vi "Create DigiPattern File_BML.vi"(7 "Timeset between frms":u32=50, 8 "error in (no error)":errorcluster, 9 "Pattern Name":string, 10 "BML Frame Array":refnum<class "BML_Frame_Root.lvclass">[](array[class]), 11 "BML_DigiPattern_Generator.lvclass":refnum<class "DigiPattern_Generator.lvclass">) -> (0 "error out":errorcluster, 3 "BML_DigiPattern_Generator.lvclass out":refnum<class "DigiPattern_Generator.lvclass">)   [LabVIEW 2018, in "DigiPattern_Generator.lvclass"]
uses:
  DigiPattern_Generator.lvclass
  BML_Frame_Root/BML_Frame_Root.lvclass
  DigiPattern_Generator.lvclass/DigiPattern_Generator.ctl
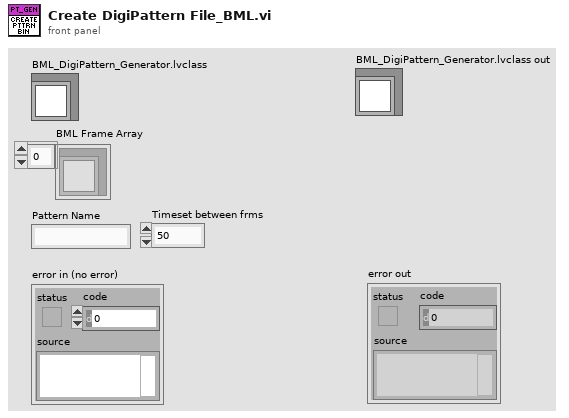
[diagram p1: front panel]
types:
  T1 = enum16{"open", "replace", "create", "open or create", "replace or create", "replace or create with confirmation"}
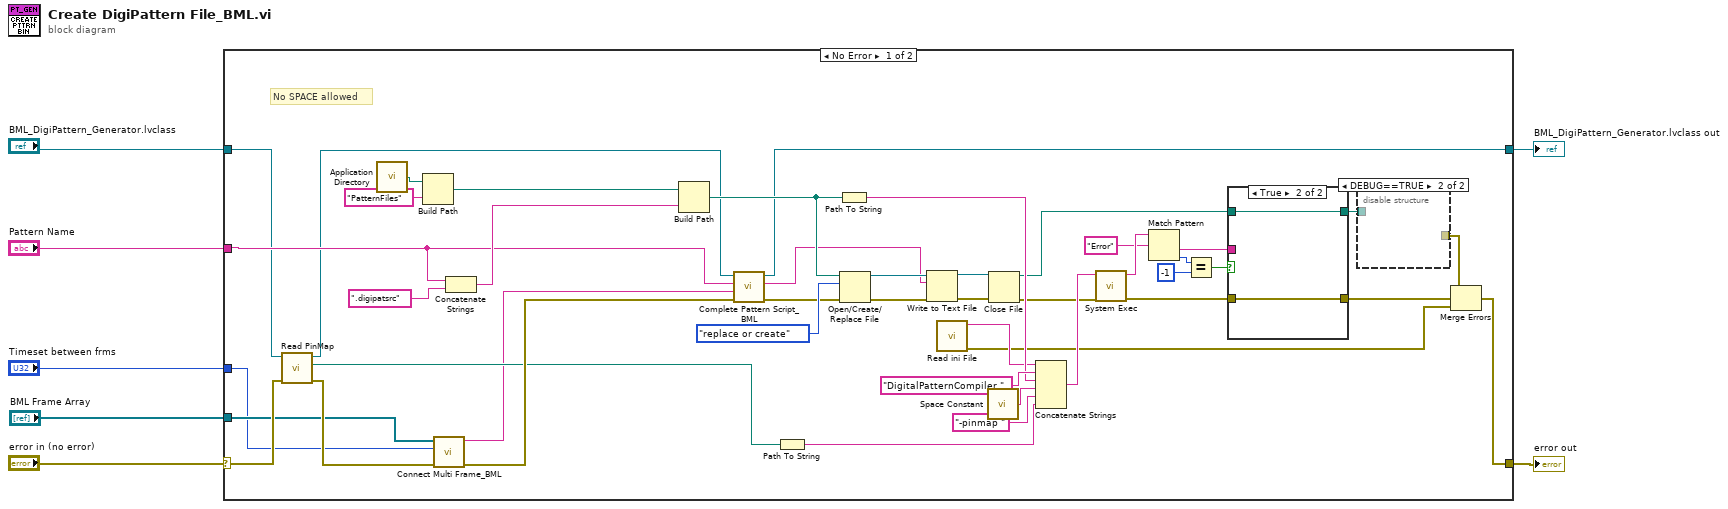
[diagram p0: block diagram]
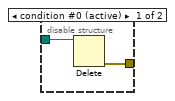
[diagram p2: hidden frame]
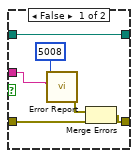
[diagram p3: hidden frame]
diagram:
  n1 = case shown="No Error" "error in (no error)" {
    selector: "error in (no error)" -> [w13 w64]
    tunnel: [w32 w64] -> w6
    tunnel: [w21 w63] -> w3
    tunnel: "BML_DigiPattern_Generator.lvclass" -> [w15 w63]
    tunnel: "Pattern Name" -> [w20 _]
    tunnel: "BML Frame Array" -> [w11 _]
    tunnel: "Timeset between frms" -> [w8 _]
    frame No Error {
      # "No SPACE allowed"
      n2 = call "Read PinMap.vi"("error in (no error)"=w13, "BML_DigiPattern_Generator in"=w15) -> ("error out"=w12:errorcluster, "PinMap"=w10:path, "BML_DigiPattern_Generator out"=w14:refnum<class "DigiPattern_Generator.lvclass">)  [unwired: 7 in]
      n3 = call <vilib>:"Application Directory.vi"() -> ("Application Directory"=w28:path)
      n4 = Build Path(base path=w28, name or relative path="PatternFiles") -> (appended path=w26:path)
      n5 = call "Connect Multi Frame_BML.vi"("error in (no error)"=w12, "Timeset between frms"=w8, "BML Frame Array"=w11) -> ("error out"=w16:errorcluster, "Connected Frame Contents"=w9:string)  [unwired: 7 in]
      n6 = Concatenate Strings(w20, ".digipatsrc" ("string")) -> (w51:string)
      n7 = Build Path(base path=w26, name or relative path=w51) -> (appended path=w46:path)
      n8 = call "Complete Pattern Script_BML.vi"("error in (no error)"=w16, "Pattern Contents"=w9, "Pattern Name"=w20, "BML_DigiPattern_Generator.lvclass"=w14) -> ("error out"=w22:errorcluster, "All Pattern Script out"=w19:string, "BML_DigiPattern_Generator.lvclass out"=w21:refnum<class "DigiPattern_Generator.lvclass">)  [unwired: 5 in]
      n9 = Path To String(path=w10) -> (string=w42:string)
      n10 = Path To String(path=w46) -> (string=w45:string)
      n11 = Open/Create/Replace File(file path (use dialog)=w46, error in=w22, operation (0:open)=T1."replace or create") -> (refnum out=w49:refnum<file>, error out=w48:errorcluster)  [unwired: 3 in, 1 out]
      n12 = Write to Text File(file (use dialog)=w49, text=w19, error in=w48) -> (refnum out=w31:refnum<file>, error out=w30:errorcluster)  [unwired: 1 in, 1 out]
      n13 = call "Read ini File.vi"() -> ("error out"=w17:errorcluster, "value"=w18:string)  [unwired: 10 in]
      n14 = call <vilib>:"Space Constant.vi"() -> ("String"=w44:string)
      n15 = Close File(refnum=w31, error in=w30) -> (path=w24:path, error out=w29:errorcluster)
      n16 = Concatenate Strings(w18, "DigitalPatternCompiler " ("string"), w45, w44, "-pinmap " ("string"), w42) -> (w41:string)
      n17 = call <vilib>:"System Exec.vi"("error in (no error)"=w29, "command line"=w41) -> ("error out"=w34:errorcluster, "standard output"=w40:string)  [unwired: 6 in, 2 out]
      n18 = Match Pattern(string=w40, regular expression="Error") -> (after substring=w35:string, offset past match=w38:i32)  [unwired: 1 in, 2 out]
      n19 = Equal?(x=w38, y=-1) -> (x = y?=w36:bool)
      n20 = case shown="True" w36 {
        tunnel: w35 -> [w56 _]
        tunnel: w34 -> [w60 w62]
        tunnel: [w59 w62] -> w33
        tunnel: w24 -> [w58 w61]
        tunnel: [w58 w61] -> w23
        frame False {
          n21 = call "Error Report.vi"("Additional info"=w56, "Error Code"=i16 5008) -> ("error out"=w55:errorcluster)  [unwired: 9 in]
          n22 = Merge Errors(w55, w60) -> (w59:errorcluster)
        }
        frame True {
        }
      }
      n23 = disable-structure shown="DEBUG==TRUE" {
        disable-tunnel: [w54 _] -> w25
        disable-tunnel: w23 -> [w53 _]
        frame condition #0 (active) {
          n24 = Delete(path (use dialog)=w53) -> (error out=w54:errorcluster)  [unwired: 4 in, 2 out]
        }
        frame condition #1 {
        }
      }
      n25 = Merge Errors(w25, w33, w17) -> (w32:errorcluster)
    }
    frame Error {
    }
  }
  "error out" <- w6
  "BML_DigiPattern_Generator.lvclass out" <- w3
